vi "PXI-Refresh AO Buffer.vi"(6 "BufferSize":i32, 8 "error in (no error)":errorcluster, 9 "AO Waveforms In":dbl[][](array[numeric]), 10 "AO Tasks":T1[](array[typedef]), 11 "Wait for buffer space? (T)":bool=TRUE) -> (0 "error out (no error)":errorcluster, 3 "AO Waveforms Out":dbl[][](array[numeric]), 4 "PauseDAQ":bool)   [LabVIEW 2020]
uses:
  Type Defs/Task Struct.ctl
  PXI Globals.vi
panel:
  out "Waveform Graph":dbl[][](graph)
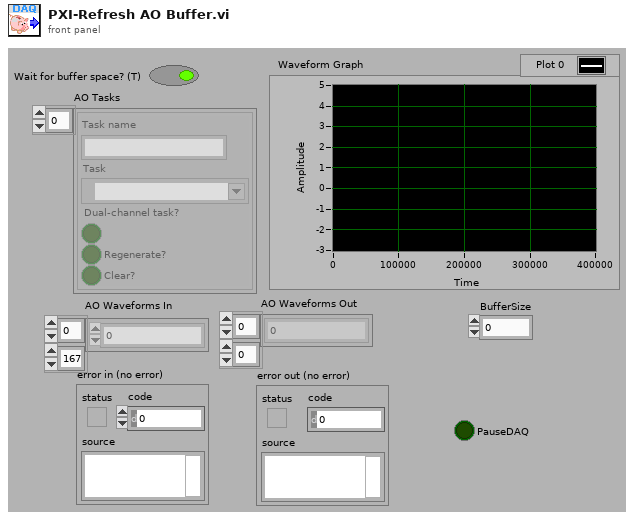
[diagram p1: front panel]
types:
  T1 = typedef "Task Struct.ctl" = cluster{"Task name":string, "Task":refnum<k21>, "Dual-channel task?":bool, "Regenerate?":bool, "Clear?":bool}
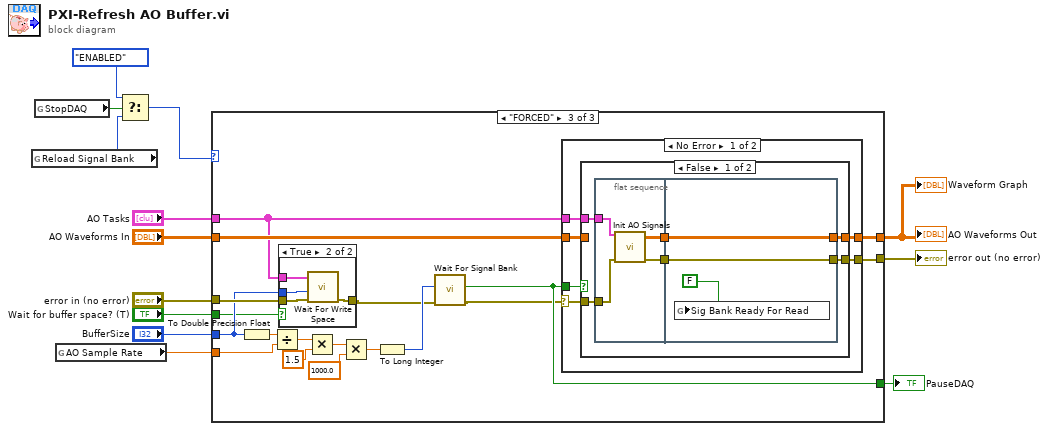
[diagram p0: block diagram]
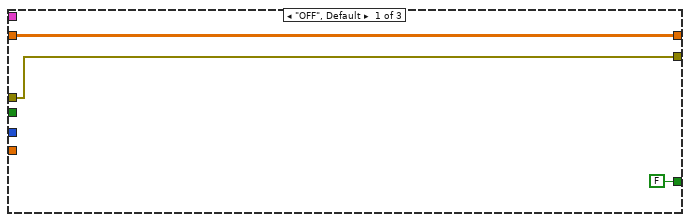
[diagram p2: hidden frame]
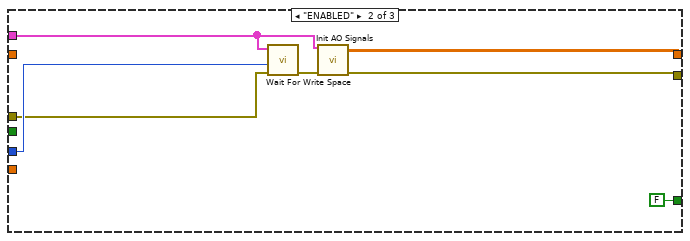
[diagram p3: hidden frame]
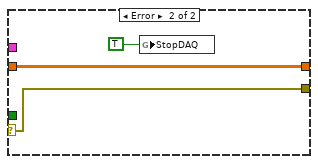
[diagram p6: hidden frame]
diagram:
  n1 = global read "PXI Globals.vi" "Reload Signal Bank"() -> (w8:enum32{"OFF", "ENABLED", "FORCED"})
  n2 = global read "PXI Globals.vi" "StopDAQ"() -> (w5:bool)
  n3 = global read "PXI Globals.vi" "AO Sample Rate"() -> (w2:dbl)
  n4 = Select(t=enum16{"OFF", "ENABLED", "FORCED"}."ENABLED", s=w5, f=w8) -> (s? t:f=w7:enum32{"OFF", "ENABLED", "FORCED"})
  n5 = case shown="\"FORCED\"" w7 {
    tunnel: "error in (no error)" -> [w16 w19 w41]
    tunnel: [w16 w22 w40] -> w12
    tunnel: "AO Waveforms In" -> [w15 _ w38]
    tunnel: [w15 w23 w39] -> w6
    tunnel: "AO Tasks" -> [_ w21 w26]
    tunnel: "BufferSize" -> [_ w20 w31]
    tunnel: [FALSE ("PauseDAQ") FALSE ("PauseDAQ") w27] -> w3
    tunnel: w2 -> [_ _ w30]
    tunnel: "Wait for buffer space? (T)" -> [_ _ w28]
    frame "OFF", Default {
    }
    frame "ENABLED" {
      n6 = call "Wait For Write Space.vi"("error in (no error)"=w19, "BufferSize"=w20, "AO Tasks"=w21) -> ("error out"=w18:errorcluster)  [unwired: 6 in, 2 out]
      n7 = call "Init AO Signals.vi"("AO Tasks"=w21, "error in (no error)"=w18) -> ("AO Waveforms"=w23:dbl[][], "error out"=w22:errorcluster)  [unwired: 12 in]
    }
    frame "FORCED" {
      n8 = To Double Precision Float(number=w31) -> (double precision float=w32:dbl)
      n9 = Divide(x=w32, y=w30) -> (x/y=w33:dbl)
      n10 = case shown="True" w28 {
        tunnel: w41 -> [w42 w46]
        tunnel: w31 -> [_ w45]
        tunnel: w26 -> [_ w44]
        tunnel: [w42 w43] -> w25
        frame False {
        }
        frame True {
          n11 = call "Wait For Write Space.vi"("error in (no error)"=w46, "BufferSize"=w45, "AO Tasks"=w44) -> ("error out"=w43:errorcluster)  [unwired: 6 in, 2 out]
        }
      }
      n12 = Multiply(x=w33, y=1.5) -> (x*y=w35:dbl)
      n13 = Multiply(x=w35, y=1000.0) -> (x*y=w37:dbl)
      n14 = To Long Integer(number=w37) -> (32bit integer=w29:i32)
      n15 = call "Wait For Signal Bank.vi"("error in (no error)"=w25, "timeout (ms)"=w29) -> ("error out"=w24:errorcluster, "PauseDAQ"=w27:bool)  [unwired: 8 in]
      n16 = case shown="No Error" w24 {
        selector: w24 -> [w50 w68]
        tunnel: [w52 w68] -> w40
        tunnel: [w51 w70] -> w39
        tunnel: w38 -> [w47 w70]
        tunnel: w26 -> [w49 _]
        tunnel: w27 -> [w48 _]
        frame No Error {
          n17 = case shown="False" w48 {
            tunnel: [w56 w67] -> w52
            tunnel: [w55 w66] -> w51
            tunnel: w50 -> [w54 w67]
            tunnel: w49 -> [w53 _]
            tunnel: w47 -> [_ w66]
            frame False {
              n18 = flat-sequence {
                tunnel: [w62] -> w58
                tunnel: [w61] -> w57
                tunnel: w54 -> [w60]
                tunnel: w53 -> [w59]
                tunnel: [w64] -> w55
                tunnel: [w65] -> w56
                tunnel: w58 -> [w65]
                tunnel: w57 -> [w64]
                frame #0 {
                  n19 = call "Init AO Signals.vi"("AO Tasks"=w59, "error in (no error)"=w60) -> ("AO Waveforms"=w61:dbl[][], "error out"=w62:errorcluster)  [unwired: 12 in]
                }
                frame #1 {
                  n20 = global write "PXI Globals.vi" "Sig Bank Ready For Read"(FALSE) -> ()
                }
              }
            }
            frame True {
            }
          }
        }
        frame Error {
          n21 = global write "PXI Globals.vi" "StopDAQ"(TRUE) -> ()
        }
      }
    }
  }
  "AO Waveforms Out" <- w6
  "error out (no error)" <- w12
  "Waveform Graph" <- w6
  "PauseDAQ" <- w3
